vi "testramp.vi"() -> ()   [LabVIEW 2015]
uses:
  BERTTA.dll
panel:
  out "return type":i32
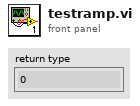
[diagram p1: front panel]
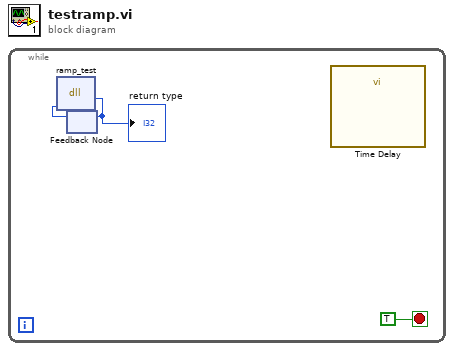
[diagram p0: block diagram]
diagram:
  n1 = while {
    stop <- TRUE stop-if-true
    n2 = feedback #1() -> (w2:i32)  [unwired: 1 in]
    n3 = dll-call lib="C:/Users/shresplab/OneDrive - Kemira Oyj/Documents/Visual Studio 2017/Projects/Bertta/BERTTA/x64/Debug/BERTTA.dll" fn="ramp_test"("last_count"=w2) -> ("return type"=w3:i32)  [unwired: 4 in, 2 out]
    "return type" <- w3
    n4 = feedback-in #1(w3) -> ()
    n5 = call "Time Delay"() -> ()  [unwired: 11 in, 1 out]
  }
